vi "Car Go Up.vi"(9 "m array":i16[][](array[numeric]), 10 "Numeric":i32, 11 "Input in":i32[][](array[numeric])) -> (2 "move or not":bool, 3 "Input out":i32[][](array[numeric]))   [LabVIEW 2021]
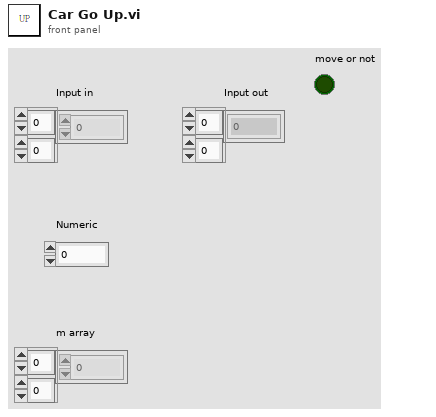
[diagram p1: front panel]
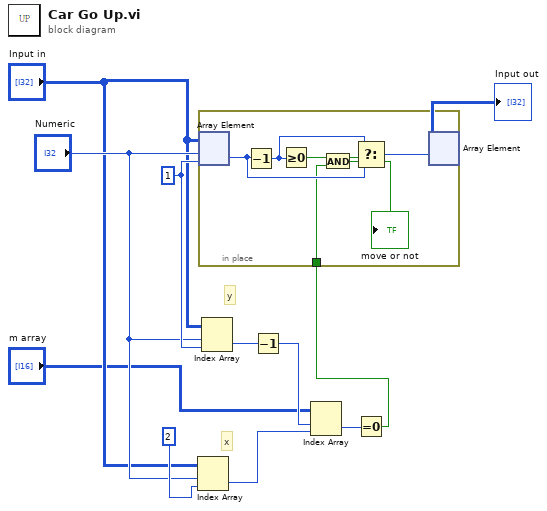
[diagram p0: block diagram]
diagram:
  w8 = 1
  # "x"
  # "y"
  n1 = Index Array(array="Input in", index (row)="Numeric", index (col)=2) -> (element=w11:i32)
  n2 = Index Array(array="Input in", index (row)="Numeric", index (col)=w8) -> (element=w4:i32)
  n3 = Decrement(x=w4) -> (x-1=w10:i32)
  n4 = Index Array(array="m array", index (row)=w10, index (col)=w11) -> (element=w3:i16)
  n5 = Equal To 0?(x=w3) -> (x = 0?=w5:bool)
  n6 = in-place {
    in-place-border: w5 -> [w12]
    n7 = in-place-array #1("Input in", "Numeric", w8) -> (w14:i32)
    n8 = Decrement(x=w14) -> (x-1=w15:i32)
    n9 = Greater Or Equal To 0?(x=w15) -> (x >= 0?=w17:bool)
    n10 = And(x=w17, y=w12) -> (x .and. y?=w13:bool)
    "move or not" <- w13
    n11 = Select(t=w15, s=w13, f=w14) -> (s? t:f=w16:i32)
    n12 = in-place-array #1(w16) -> (→"Input out":i32[][])  [unwired: 2 out]
  }
